vi "ADFX_Do_Button_Ctrl_Changed.vi"(0 "Data in":T2, 5 "Trigger Type:":T1(ring), 7 "New Sound Files":path[](array[path]), 9 "Old Sound Files":path[](array[path]), 11 "error in (no error)":errorcluster) -> (4 "Data out":T2, 15 "error out":errorcluster)   [LabVIEW 2015]
uses:
  controls/AFXP Data.ctl
  controls/AFCP Setup.ctl
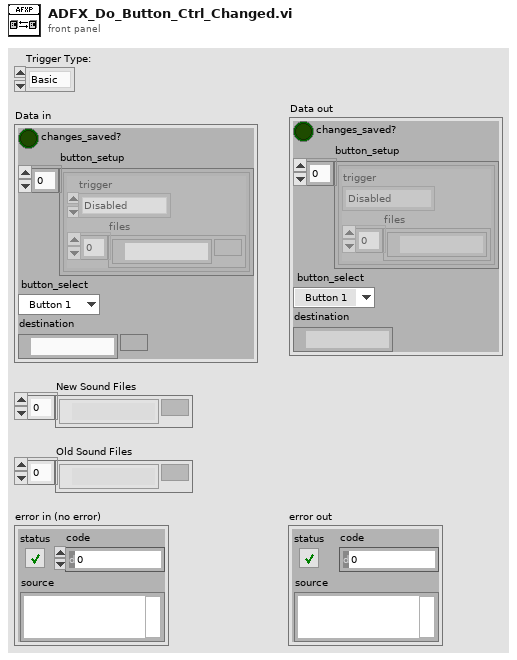
[diagram p1: front panel]
types:
  T1 = enum16{"Basic", "Hold-Loop", "Latch-Loop", "Next", "Random", "Disabled"}
  T2 = typedef "AFXP Data.ctl" = cluster{"changes_saved?":bool, "button_setup":T3[], "button_select":enum8{"Button 1", "Button 2", "Button 3", "Button 4", "Button 5", "Button 6", "Button 7", "Button 8", "Button 9", "Button 10", "Button 11", "Button 12"}, "destination":path}
  T3 = typedef "AFCP Setup.ctl" = cluster{"trigger":enum16{"Basic", "Hold-Loop", "Latch-Loop", "Next", "Random", "Disabled"}, "files":path[]}
  T4 = enum8{"Button 1", "Button 2", "Button 3", "Button 4", "Button 5", "Button 6", "Button 7", "Button 8", "Button 9", "Button 10", "Button 11", "Button 12"}
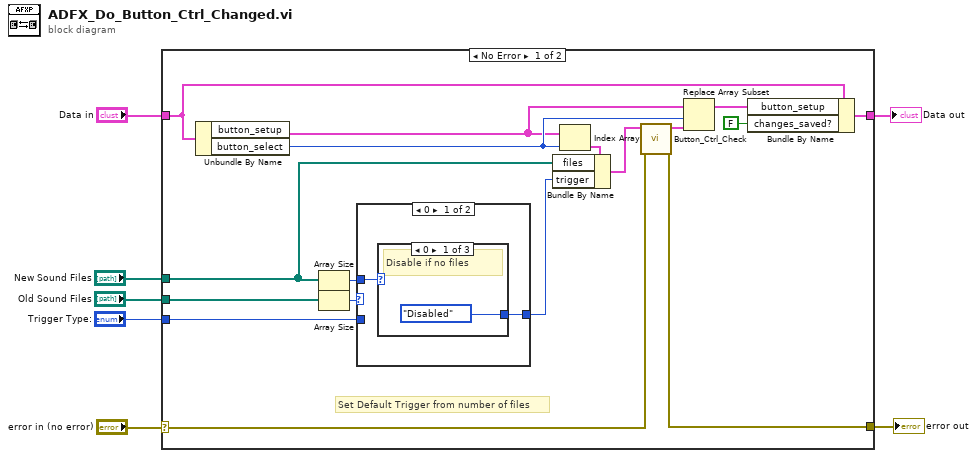
[diagram p0: block diagram]
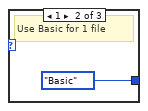
[diagram p2: hidden frame]
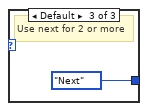
[diagram p3: hidden frame]
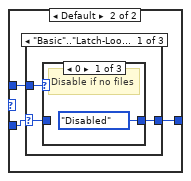
[diagram p4: hidden frame]
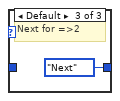
[diagram p6: hidden frame]
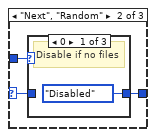
[diagram p7: hidden frame]
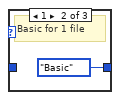
[diagram p8: hidden frame]
diagram:
  n1 = case shown="No Error" "error in (no error)" {
    selector: "error in (no error)" -> [w24 w47]
    tunnel: "New Sound Files" -> [w20 _]
    tunnel: [w15 w46] -> w6
    tunnel: "Data in" -> [w8 w46]
    tunnel: "Trigger Type:" -> [w14 _]
    tunnel: "Old Sound Files" -> [w11 _]
    tunnel: [w10 w47] -> w2
    frame No Error {
      # "Set Default Trigger from number of files"
      n2 = Unbundle By Name(w8) -> ("button_setup"=w16:T3[], "button_select"=w18:T4)
      n3 = Array Size(array=w20) -> (size(s)=w13:i32)
      n4 = Array Size(array=w11) -> (size(s)=w12:i32)
      n5 = case shown="0" w12 {
        tunnel: w13 -> [w26 w32]
        tunnel: w14 -> [_ w31]
        tunnel: [w25 w30] -> w19
        frame 0 {
          n6 = case shown="0" w26 {
            tunnel: [T1."Disabled" ("Trigger Type") T1."Basic" ("Trigger Type") T1."Next" ("Trigger Type")] -> w25
            frame 0 {
              # "Disable if no files"
            }
            frame 1 {
              # "Use Basic for 1 file"
            }
            frame Default {
              # "Use next for 2 or more"
            }
          }
        }
        frame Default {
          n7 = case shown="\"Basic\"..\"Latch-Loop\"" w31 {
            selector: w31 -> [w33 w39 w45]
            tunnel: [w34 w40 w45] -> w30
            tunnel: w32 -> [w35 w41 _]
            frame "Basic".."Latch-Loop" {
              n8 = case shown="0" w35 {
                tunnel: [T1."Disabled" ("Trigger Type") w37 T1."Next" ("Trigger Type")] -> w34
                tunnel: w33 -> [_ w37 _]
                frame 0 {
                  # "Disable if no files"
                }
                frame 1 {
                  # "No change for 1 file"
                }
                frame Default {
                  # "Next for =>2"
                }
              }
            }
            frame "Next", "Random" {
              n9 = case shown="0" w41 {
                tunnel: [T1."Disabled" ("Trigger Type") T1."Basic" ("Trigger Type") w44] -> w40
                tunnel: w39 -> [_ _ w44]
                frame 0 {
                  # "Disable if no files"
                }
                frame 1 {
                  # "Basic for 1 file"
                }
                frame Default {
                  # "No change if 2 or more files"
                }
              }
            }
            frame "Disabled" {
            }
          }
        }
      }
      n10 = Index Array(array=w16, index=w18) -> (element=w23:T3)
      n11 = Bundle By Name(cluster=w23, "files"=w20, "trigger"=w19) -> (w21:T3)
      n12 = call "Button_Ctrl_Check.vi"("error in (no error)"=w24, "Button Ctrl in"=w21) -> ("error out"=w10:errorcluster, "Button Ctrl out"=w22:T3)  [unwired: 8 in]
      n13 = Replace Array Subset(array=w16, new element=w22, index=w18) -> (w17:T3[])
      n14 = Bundle By Name(cluster=w8, "button_setup"=w17, "changes_saved?"=FALSE) -> (w15:T2)
    }
    frame Error {
    }
  }
  "Data out" <- w6
  "error out" <- w2
